vi "Set Function Between Channels.vi"(6 "Operator":u16(ring) items=["Add", "Substract", "Multiply", "Divide"], 8 "error in (no error)":errorcluster, 9 "Channel Y":u16(ring) items=["A1"=0, "A2"=1, "A3"=2, "A4"=3, "A5"=4, "A6"=5, "A7"=6, "A8"=7, "A9"=8, "A10"=9, "K1"=200, "K2"=201, "K3"=202, "K4"=203, "FA1"=204, "FA2"=205, "FA3"=206, "FA4"=207], 10 "Channel X":u16(ring) items=["A1"=0, "A2"=1, "A3"=2, "A4"=3, "A5"=4, "A6"=5, "A7"=6, "A8"=7, "A9"=8, "A10"=9, "K1"=200, "K2"=201, "K3"=202, "K4"=203, "FA1"=204, "FA2"=205, "FA3"=206, "FA4"=207], 11 "VISA resource name":refnum<visa-resource-name>) -> (0 "error out":errorcluster, 3 "VISA resource name out":refnum<visa-resource-name>)   [LabVIEW 2017, in "Sefram DAS220.lvlib"]
doc: "Setup a function between channel (from FA1 to FJ4) to apply aX2+bY+c with X the channel X selected and Y the channel Y selected.\nFor example : a (A1)2+bA5+c"
uses:
  <instrlib>/Sefram DAS220/Sefram DAS220.lvlib
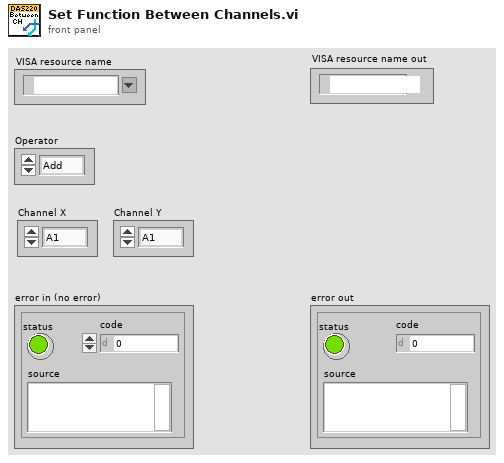
[diagram p1: front panel]
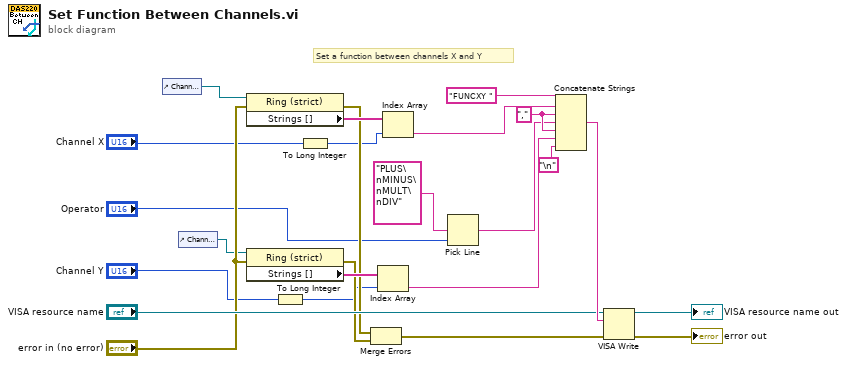
[diagram p0: block diagram]
diagram:
  w15 = "," ("string")
  # "Set a function between channels X and Y"
  n1 = control-ref of="Channel X"() -> (w3:refnum<vi>)
  n2 = control-ref of="Channel Y"() -> (w1:refnum<vi>)
  n3 = property class="Ring (strict)"(reference=w3, error in="error in (no error)") -> (error out=w9:errorcluster, "Strings []"=w19:string[])  [unwired: 1 out]
  n4 = property class="Ring (strict)"(reference=w1, error in="error in (no error)") -> (error out=w8:errorcluster, "Strings []"=w18:string[])  [unwired: 1 out]
  n5 = To Long Integer(number="Channel Y") -> (32bit integer=w6:i32)
  n6 = To Long Integer(number="Channel X") -> (32bit integer=w7:i32)
  n7 = Merge Errors(w9, w8) -> (w10:errorcluster)
  n8 = Index Array(array=w18, index=w6) -> (element=w13:string)
  n9 = Index Array(array=w19, index=w7) -> (element=w17:string)
  n10 = Pick Line(multi-line string="PLUS\nMINUS\nMULT\nDIV", line index="Operator") -> (output string=w14:string)  [unwired: 1 in]
  n11 = Concatenate Strings("FUNCXY " ("string"), w17, w15, w14, w15, w13, "\n") -> (w24:string)
  n12 = VISA Write(VISA resource name="VISA resource name", write buffer=w24, error in (no error)=w10) -> (VISA resource name out=→"VISA resource name out":refnum<visa-resource-name>, error out=→"error out":errorcluster)  [unwired: 1 out]
